vi "Step LUT.vi"(11 "Step Name":string) -> (2 "Available Steps":string[](array[string]), 3 "Relative Path":path)   [LabVIEW 2018]
doc: "This VI contains a Look Up Table (LUT) that includes the names of all the control steps and their relative paths on disk. This LUT needs to be updated every time a control step is added or removed.\nIf a control step name is connected as an input, the path to the configuration VI for that step is returned in the 'Relative Path' terminal."
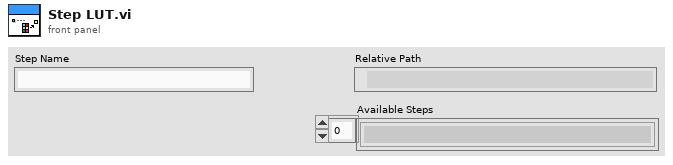
[diagram p1: front panel]
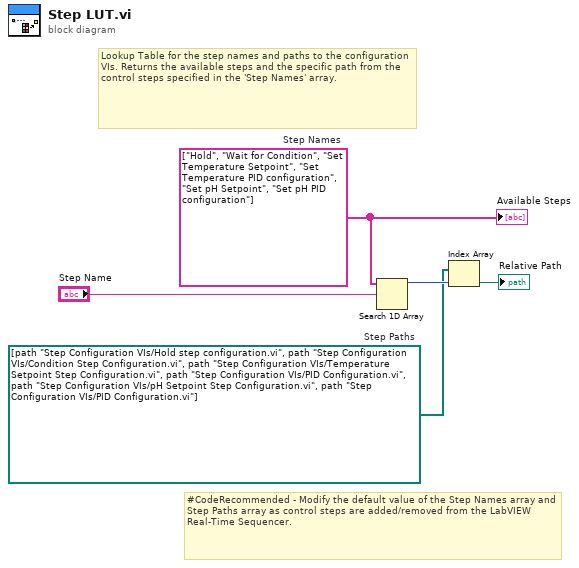
[diagram p0: block diagram]
diagram:
  w1 = path[] [path "Step Configuration VIs/Hold step configuration.vi", path "Step Configuration VIs/Condition Step Configuration.vi", path "Step Configuration VIs/Temperature Setpoint Step Configuration.vi", path "Step Configuration VIs/PID Configuration.vi", path "Step Configuration VIs/pH Setpoint Step Configuration.vi", path "Step Configuration VIs/PID Configuration.vi"]  # Step Paths
  w2 = string[] ["Hold", "Wait for Condition", "Set Temperature Setpoint", "Set Temperature PID configuration", "Set pH Setpoint", "Set pH PID configuration"]  # Step Names
  # "#CodeRecommended - Modify the default value of the Step Names array and Step Paths array as control steps are added/removed from the LabVIEW Real-Time Sequencer."
  # "Lookup Table for the step names and paths to the configuration VIs. Returns the available steps and the specific path from the control steps specified in the 'Step Names' array."
  n1 = Search 1D Array(1D array=w2, element="Step Name") -> (index of element=w3:i32)  [unwired: 1 in]
  n2 = Index Array(array=w1, index=w3) -> (element=→"Relative Path":path)
  "Available Steps" <- w2
